vi "Get Relation.vi"(11 "Sender in":refnum<class "Sender.lvclass">) -> (2 "Relation":T1)   [LabVIEW 2021, in "jettl.lvlib" / "Sender.lvlib" / "Sender.lvclass"]
uses:
  Sender.lvclass
  Relation.ctl
  Sender.lvlib
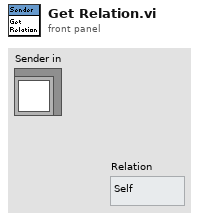
[diagram p1: front panel]
types:
  T1 = typedef "jettl.lvlib/Sender.lvlib/Relation.ctl" = enum16{"Self", "Creator", "Created"}
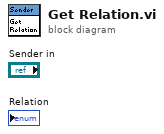
[diagram p0: block diagram]
diagram:
